vi "Facade.vi"(0 "Data In":T5, 2 "Display State In":T3, 3 "Container State":T4) -> (6 "Data Out":T5, 7 "Display State Out":T3, 8 "Action":T2)   [LabVIEW 2020, in "Waveform.xctl"]
uses:
  Waveform.xctl
  Data.vi
  Classes/Waveforms/Waveform/Waveform.lvclass
  D:/Development/epl-vi-lib/Koop/KObject Class/KObject.lvclass
  <vilib>/_xctls/Container State.ctl
  State.vi
  <vilib>/_xctls/Action.ctl
  Tone/Tone.xctl
  Classes/Waveforms/Tone/Tone.lvclass
  D:/Development/epl-vi-lib/Signal Synthesis VIs/4th Generation/Classes/Waveforms/Waveform/Waveform.lvclass
  Noise/Noise.xctl
  Classes/Waveforms/Noise/Noise.lvclass
  Tone Cloud/ToneCloud.xctl
  Classes/Waveforms/Tone Cloud/Tone Cloud.lvclass
  File/File.xctl
  Classes/Waveforms/File/File.lvclass
  FM Sweep/FM Sweep.xctl
  Classes/Waveforms/FM Sweep/FM Sweep.lvclass
  Pulse Train/Pulse Train.xctl
  Classes/Waveforms/Pulse Train/Pulse Train.lvclass
  Moving Ripple Noise/Moving Ripple Noise.xctl
  Classes/Waveforms/Moving Ripple Noise/Moving Ripple Noise.lvclass
  <vilib>/_xctls/XControlSupport.lvlib
  Koop/KObject Class/KObject.lvclass
panel:
  in  "Tabs":T1(tab)
  in  "File":refnum<class "File.lvclass">(xcontrol)
  in  "FM Sweep":refnum<class "FM Sweep.lvclass">(xcontrol)
  in  "Moving Ripple Noise":refnum<class "Moving Ripple Noise.lvclass">(xcontrol)
  in  "Noise":refnum<class "Noise.lvclass">(xcontrol)
  in  "Pulse Train":refnum<class "Pulse Train.lvclass">(xcontrol)
  in  "Tone":refnum<class "Tone.lvclass">(xcontrol)=refnum
  in  "Tone Cloud":refnum<class "Tone Cloud.lvclass">(xcontrol)
  in  "Shape":u16(ring) items=["OFF", "File", "FM Sweep", "Moving Ripple Noise", "Noise", "Pulse Train", "Tone", "Tone Cloud"]
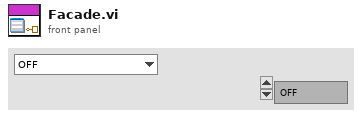
[diagram p1: front panel]
types:
  T1 = enum32{"OFF", "File", "FM Sweep", "Moving Ripple Noise", "Noise", "Pulse Train", "Tone", "Tone Cloud"}
  T2 = typedef "XControlSupport.lvlib/Action.ctl" = cluster{"Data Changed?":bool, "State Changed?":bool, "Action Name":string}
  T3 = typedef "Waveform.xctl/State.vi" = cluster{"action":string}
  T4 = typedef "XControlSupport.lvlib/Container State.ctl" = cluster{"Indicator?":bool, "Run Mode?":bool, " Refnum":refnum<vi>}
  T5 = typedef "Waveform.xctl/Data.vi" = refnum<class "Waveform.lvclass">
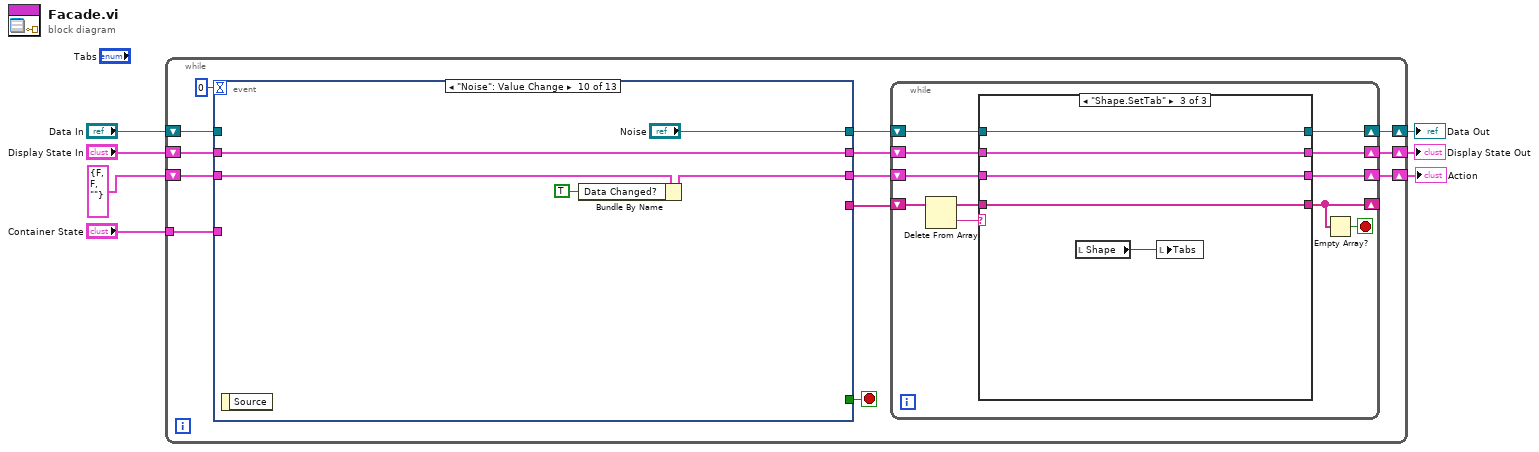
[diagram p0: block diagram]
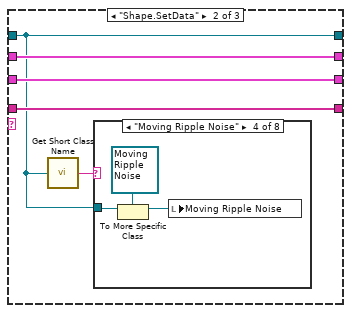
[diagram p3: hidden frame]
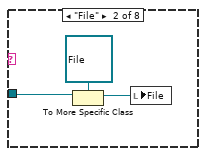
[diagram p5: hidden frame]
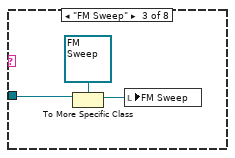
[diagram p6: hidden frame]
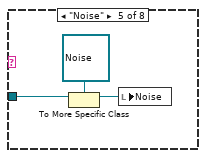
[diagram p7: hidden frame]
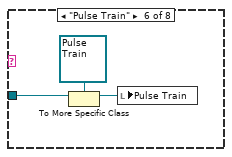
[diagram p8: hidden frame]
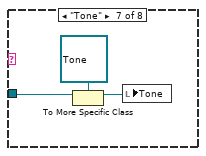
[diagram p9: hidden frame]
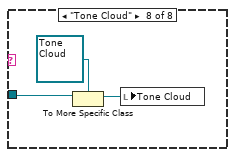
[diagram p10: hidden frame]
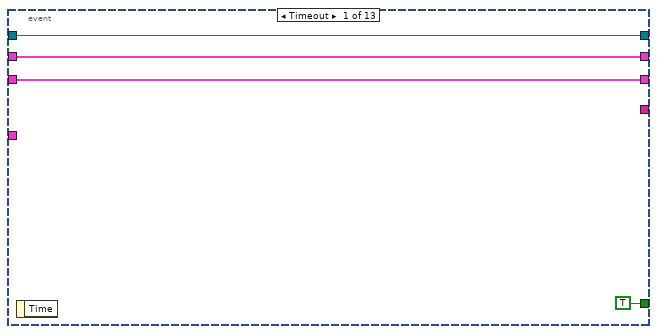
[diagram p11: hidden frame]
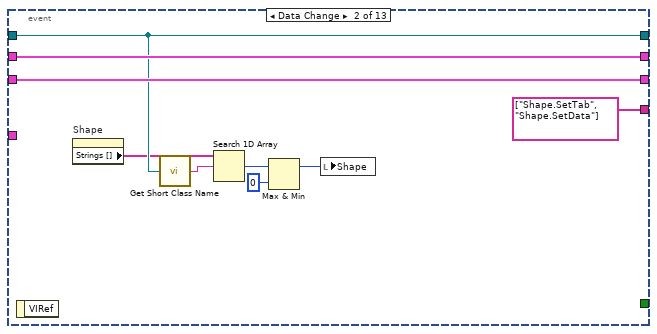
[diagram p12: hidden frame]
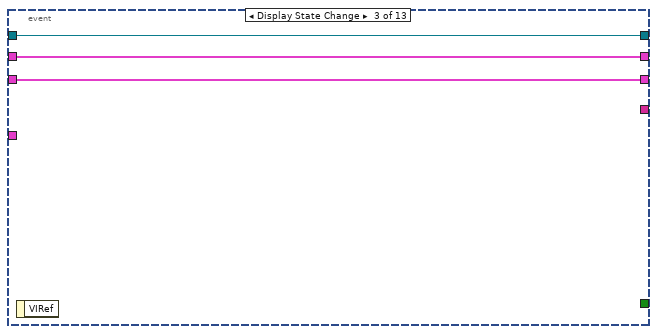
[diagram p13: hidden frame]
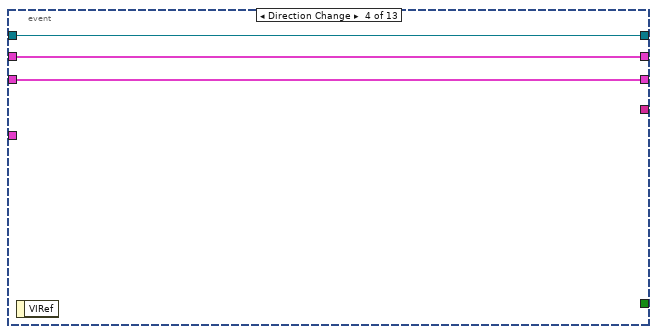
[diagram p14: hidden frame]
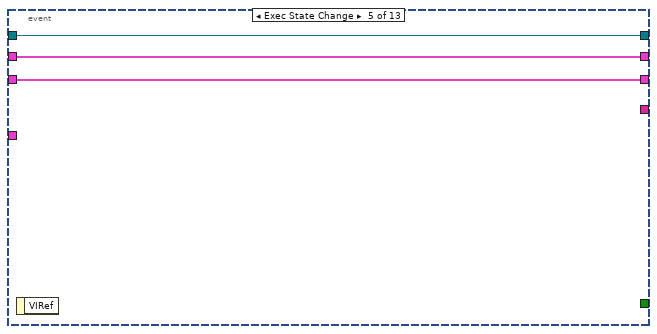
[diagram p15: hidden frame]
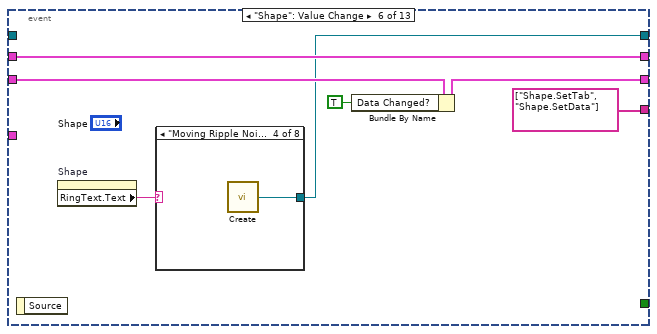
[diagram p16: hidden frame]
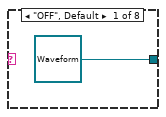
[diagram p17: hidden frame]
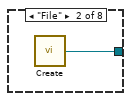
[diagram p18: hidden frame]
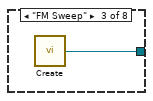
[diagram p19: hidden frame]
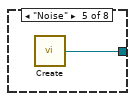
[diagram p20: hidden frame]
diagram:
  n1 = while {
    shift-right: [w8] -> w4
    shift-left: "Display State In" -> [w20]
    tunnel: "Container State" -> [w17]
    shift-right: [w10] -> w7
    shift-left: "Data In" -> [w16]
    shift-right: [w9] -> w2
    shift-left: T2 {"Data Changed?"=FALSE, "State Changed?"=FALSE, "Action Name"=""} ("Action") -> [w15]
    stop <- w19 stop-if-true
    n2 = event shown="[9] \"Noise\": Value Change" {
      selector: _ -> [_ _ _ _ _ _ _ _ _ _ _ _ _]
      dyn-events: _ -> [_ _ _ _ _ _ _ _ _ _ _ _ _]
      timeout: 0 -> [_ _ _ _ _ _ _ _ _ _ _ _ _]
      tunnel: w20 -> [w68 w79 w82 w85 w88 w95 w108 w113 w118 w123 w128 w133 w138]
      tunnel: [w68 w79 w82 w85 w88 w95 w108 w113 w118 w123 w128 w133 w138] -> w12
      tunnel: [TRUE _ _ _ _ _ _ _ _ _ _ _ _] -> w19
      tunnel: w17 -> [_ _ _ _ _ _ _ _ _ _ _ _ _]
      tunnel: w16 -> [w67 w76 w81 w84 w87 _ _ _ _ _ _ _ _]
      tunnel: [w67 w76 w81 w84 w87 w89 "File" "FM Sweep" "Moving Ripple Noise" "Noise" "Pulse Train" "Tone" "Tone Cloud"] -> w13
      tunnel: [w69 w78 w80 w83 w86 w92 w106 w111 w116 w121 w126 w130 w136] -> w11
      tunnel: w15 -> [w69 w78 w80 w83 w86 w94 w107 w112 w117 w122 w127 w132 w137]
      tunnel: [_ string[] ["Shape.SetTab", "Shape.SetData"] _ _ _ string[] ["Shape.SetTab", "Shape.SetData"] _ _ _ _ _ _ _] -> w14
      event Timeout {
        n3 = event-data() -> ()  [unwired: 1 in, 1 out]
      }
      event Data Change {
        n4 = event-data() -> ()  [unwired: 1 in, 1 out]
        n5 = property on="Shape" class="Ring (strict)"() -> ("Strings []"=w75:string[])  [unwired: 2 in, 2 out]
        n6 = call "Get Short Class Name.vi"("KObject in"=w76) -> ("Class"=w74:string)  [unwired: 4 in]
        n7 = Search 1D Array(1D array=w75, element=w74) -> (index of element=w73:i32)  [unwired: 1 in]
        n8 = Max & Min(x=w73, y=0) -> (max(x,y)=w71:i32)  [unwired: 1 out]
        n9 = local write "Shape"(w71) -> ()
      }
      event Display State Change {
        n10 = event-data() -> ()  [unwired: 1 in, 1 out]
      }
      event Direction Change {
        n11 = event-data() -> ()  [unwired: 1 in, 1 out]
      }
      event Exec State Change {
        n12 = event-data() -> ()  [unwired: 1 in, 1 out]
      }
      event "Shape": Value Change {
        n13 = event-data() -> ()  [unwired: 1 in, 1 out]
        n14 = property on="Shape" class="Ring (strict)"() -> ("RingText.Text"=w90:string)  [unwired: 2 in, 2 out]
        n15 = case shown="\"Moving Ripple Noise\"" w90 {
          tunnel: [refnum<class "Waveform.lvclass"> refnum ("Waveform") w97 w98 w99 w100 w101 w102 w103] -> w89
          frame "OFF", Default {
          }
          frame "File" {
            n16 = call "Create.vi"() -> ("File"=w97:refnum<class "File.lvclass">)  [unwired: 15 in]
          }
          frame "FM Sweep" {
            n17 = call "Create.vi"() -> ("FM Sweep"=w98:refnum<class "FM Sweep.lvclass">)  [unwired: 15 in]
          }
          frame "Moving Ripple Noise" {
            n18 = call "Create.vi"() -> ("Moving Ripple Noise"=w99:refnum<class "Moving Ripple Noise.lvclass">)  [unwired: 15 in]
          }
          frame "Noise" {
            n19 = call "Create.vi"() -> ("Noise"=w100:refnum<class "Noise.lvclass">)  [unwired: 15 in]
          }
          frame "Pulse Train" {
            n20 = call "Create.vi"() -> ("Pulse Train"=w101:refnum<class "Pulse Train.lvclass">)  [unwired: 15 in]
          }
          frame "Tone" {
            n21 = call "Create.vi"() -> ("Tone"=w102:refnum<class "Tone.lvclass">)  [unwired: 15 in]
          }
          frame "Tone Cloud" {
            n22 = call "Create.vi"() -> ("ToneCloud"=w103:refnum<class "Tone Cloud.lvclass">)  [unwired: 15 in]
          }
        }
        n23 = Bundle By Name(cluster=w94, "Data Changed?"=TRUE) -> (w92:T2)
      }
      event "File": Value Change {
        n24 = event-data() -> ()  [unwired: 1 in, 1 out]
        n25 = Bundle By Name(cluster=w107, "Data Changed?"=TRUE) -> (w106:T2)
      }
      event "FM Sweep": Value Change {
        n26 = event-data() -> ()  [unwired: 1 in, 1 out]
        n27 = Bundle By Name(cluster=w112, "Data Changed?"=TRUE) -> (w111:T2)
      }
      event "Moving Ripple Noise": Value Change {
        n28 = event-data() -> ()  [unwired: 1 in, 1 out]
        n29 = Bundle By Name(cluster=w117, "Data Changed?"=TRUE) -> (w116:T2)
      }
      event "Noise": Value Change {
        n30 = event-data() -> ()  [unwired: 1 in, 1 out]
        n31 = Bundle By Name(cluster=w122, "Data Changed?"=TRUE) -> (w121:T2)
      }
      event "Pulse Train": Value Change {
        n32 = event-data() -> ()  [unwired: 1 in, 1 out]
        n33 = Bundle By Name(cluster=w127, "Data Changed?"=TRUE) -> (w126:T2)
      }
      event "Tone": Value Change {
        n34 = event-data() -> ()  [unwired: 1 in, 1 out]
        n35 = Bundle By Name(cluster=w132, "Data Changed?"=TRUE) -> (w130:T2)
      }
      event "Tone Cloud": Value Change {
        n36 = event-data() -> ()  [unwired: 1 in, 1 out]
        n37 = Bundle By Name(cluster=w137, "Data Changed?"=TRUE) -> (w136:T2)
      }
    }
    n38 = while {
      shift-right: [w28] -> _
      shift-left: w14 -> [w31]
      shift-right: [w23] -> w10
      shift-left: w13 -> [w26]
      shift-right: [w22] -> w8
      shift-left: w12 -> [w25]
      shift-right: [w21] -> w9
      shift-left: w11 -> [w24]
      stop <- w27 stop-if-true
      n39 = Delete From Array(array=w31) -> (deleted portion=w29:string, array with subset deleted=w30:string[])  [unwired: 2 in]
      n40 = case shown="\"Shape.SetTab\"" w29 {
        tunnel: w30 -> [w35 w40 w66]
        tunnel: [w35 w40 w66] -> w28
        tunnel: w26 -> [w34 w36 w65]
        tunnel: w25 -> [w33 w39 w64]
        tunnel: w24 -> [w32 w38 w63]
        tunnel: [w34 w36 w65] -> w23
        tunnel: [w33 w39 w64] -> w22
        tunnel: [w32 w38 w63] -> w21
        frame "", Default {
        }
        frame "Shape.SetData" {
          n41 = call "Get Short Class Name.vi"("KObject in"=w36) -> ("Class"=w37:string)  [unwired: 4 in]
          n42 = case shown="\"Moving Ripple Noise\"" w37 {
            tunnel: w36 -> [_ w43 w46 w49 w52 w55 w58 w61]
            frame "OFF", Default {
            }
            frame "File" {
              n43 = To More Specific Class(target class=refnum<class "File.lvclass"> refnum ("File"), reference=w43) -> (specific class reference=w42:refnum<class "File.lvclass">)  [unwired: 1 in, 1 out]
              n44 = local write "File"(w42) -> ()
            }
            frame "FM Sweep" {
              n45 = To More Specific Class(target class=refnum<class "FM Sweep.lvclass"> refnum ("FM Sweep"), reference=w46) -> (specific class reference=w45:refnum<class "FM Sweep.lvclass">)  [unwired: 1 in, 1 out]
              n46 = local write "FM Sweep"(w45) -> ()
            }
            frame "Moving Ripple Noise" {
              n47 = To More Specific Class(target class=refnum<class "Moving Ripple Noise.lvclass"> refnum ("MRN"), reference=w49) -> (specific class reference=w48:refnum<class "Moving Ripple Noise.lvclass">)  [unwired: 1 in, 1 out]
              n48 = local write "Moving Ripple Noise"(w48) -> ()
            }
            frame "Noise" {
              n49 = To More Specific Class(target class=refnum<class "Noise.lvclass"> refnum ("Noise"), reference=w52) -> (specific class reference=w50:refnum<class "Noise.lvclass">)  [unwired: 1 in, 1 out]
              n50 = local write "Noise"(w50) -> ()
            }
            frame "Pulse Train" {
              n51 = To More Specific Class(target class=refnum<class "Pulse Train.lvclass"> refnum ("Pulse Train"), reference=w55) -> (specific class reference=w53:refnum<class "Pulse Train.lvclass">)  [unwired: 1 in, 1 out]
              n52 = local write "Pulse Train"(w53) -> ()
            }
            frame "Tone" {
              n53 = To More Specific Class(target class=refnum<class "Tone.lvclass"> refnum ("Tone"), reference=w58) -> (specific class reference=w57:refnum<class "Tone.lvclass">)  [unwired: 1 in, 1 out]
              n54 = local write "Tone"(w57) -> ()
            }
            frame "Tone Cloud" {
              n55 = To More Specific Class(target class=refnum<class "Tone Cloud.lvclass"> refnum ("ToneCloud"), reference=w61) -> (specific class reference=w60:refnum<class "Tone Cloud.lvclass">)  [unwired: 1 in, 1 out]
              n56 = local write "Tone Cloud"(w60) -> ()
            }
          }
        }
        frame "Shape.SetTab" {
          n57 = local read "Shape"() -> (w62:u16)
          n58 = local write "Tabs"(w62) -> ()
        }
      }
      n59 = Empty Array?(array=w28) -> (empty?=w27:bool)
    }
  }
  "Display State Out" <- w4
  "Data Out" <- w7
  "Action" <- w2
